vi "Get Specified FP Objects.vi"(8 "error in":errorcluster, 9 "Secondary Data":variant, 10 "Object Type":T1(ring)=enum."Generic", 11 "Diagram In":refnum<vi>) -> (0 "error out":errorcluster, 2 "All Objects":refnum<vi>[](array[refnum]), 3 "Diagram Out":refnum<vi>)   [LabVIEW 2012, in "Scripting Tools.lvlib"]
doc: "Returns all GObjects from the block diagram referenced by <B>Diagram In</B>, including all those in sub-diagrams (loops and sequence structures etc)."
uses:
  Scripting Tools.lvlib
  <vilib>/Utility/traverseref.llb/TRef TravTarget.ctl
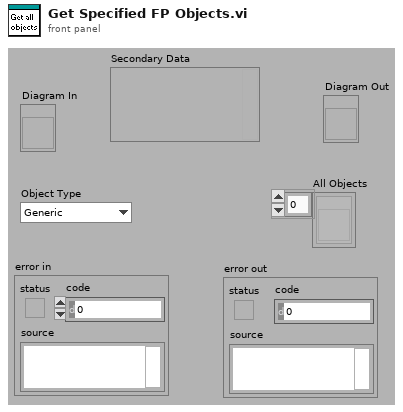
[diagram p1: front panel]
types:
  T1 = enum16{"Application", "VI", "PolymorphicVI", "MethodVI", "FacadeVI", "Generic", "FlatSequenceFrame", "TimeSequenceFrame", "SubWizard", "CodeWizard", "StateDiagramWizard", "MasterWizard", "Probe", "ConnectorPane", "Page", "Cursor", "Plot", "GObject", "TimedStructDCO", "SynchronousDataFlowDCO", "PolymorphicVISelector", "FlatSequenceOuterTunnel", "FlatSequenceInnerTunnel", "SimulationDCO", "FlatSequence", "TimeFlatSequence", "PropertyItem", "Wire", "SequenceLocal", "Tunnel", "SelectorTunnel", "LeftShiftRegister", "LoopTunnel", "RightShiftRegister", "Node", "TimedSequence", "XNode", "XDataNode", "StaticVIReference", "ControlReferenceConstant", "GrowableFunction", "Unbundler", "NamedUnbundler", "FormatScanString", "ObjectFunction", "Constructor", "Invoke", "Property", "CallLibrary", "CIN", "Bundler", "NamedBundler", "BuildArray", "IndexArray", "CompoundArithmetic", "BuildClusterArray", "Formula", "MathScriptNode", "ScriptNode", "Structure", "SynchronousDataFlowNode", "SimulationNode", "MultiFrameStructure", "DisableStructure", "EventStructure", "CaseStructure", "Sequence", "ExternalNode", "Loop", "WhileLoop", "TimedLoop", "ForLoop", "UnitCast", "CallByRef", "SubVI", "ConfNode", "PolymorphicSubVI", "Function", "FileDialog", "ArrayToCluster", "GPIBReadWrite", "FlattenUnflattenString", "FlattenString", "TypeCast", "ReadWriteFile", "Comparison", "Local", "Global", "FormulaParameter", "MathScriptNodeParameter", "ScriptNodeParameter", "Constant", "LabVIEWClassConstant", "AbsTimeConstant", "RefNumConstant", "ClassSpecifierConstant", "ColorBoxConstant", "IONameConstant", "GenClassTagFlatRefConstant", "GenClassTagRefConstant", "DAQmxNameConstant", "IVILogicalNameConstant", "VISAResourceNameConstant", "DAQChannelNameConstant", "DSCTagConstant", "BooleanConstant", "FixedConstant", "ClusterConstant", "StringConstant", "ComboBoxConstant", "NumericConstant", "NamedNumericConstant", "EnumConstant", "RingConstant", "DigitalNumericConstant", "ArrayConstant", "PathConstant", "Terminal", "OuterTerminal", "InnerTerminal", "ControlTerminal", "AbstractDiagram", "MathDiagram", "Diagram", "SDFCompanionDiagram", "SdfDiagram", "CompanionDiagram", "SimDiagram", "TopLevelDiagram", "Splitter", "Pane", "Scale", "SlideScale", "ColorGraphScale", "GraphScale", "ColorScale", "RotaryColorScale", "Panel", "Control", "LabVIEWClassControl", "SceneGraphDisplay", "Scrollbar", "Pixmap", "PlugInDDODummyContainer", "PlugInControl", "TreeControl", "SubPanel", "DigitalTable", "AbsTime", "PageSelector", "TabControl", "WaveformData", "MulticolumnListbox", "Cluster", "RadioButtonsControl", "IOName", "GenClassTagFlatRef", "GenClassTagRef", "DAQmxName", "IVILogicalName", "VISAResourceName", "DAQChannelName", "DSCTag", "String", "ComboBox", "GraphChart", "MixedSignalGraph", "IntensityGraph", "IntensityChart", "WaveformGraph", "DigitalGraph", "XYGraph", "WaveformChart", "Numeric", "NumericWithScale", "Knob", "Slide", "ColorRamp", "NamedNumeric", "Enum", "Ring", "Digital", "ActiveXContainer", "Picture", "Array", "Table", "ListBox", "Path", "LVVariant", "RefNum", "GenClassRef", "LVObjectRefNum", "VIRefNum", "TypedRefNum", "Boolean", "ColorBox", "Decoration", "Text", "NumericText", "Project", "ProjectItem", "PropertyFolder", "XPropertyFolder", "TargetItem", "Library", "XInterfaceLibrary", "XNodeLibrary", "XControlLibrary", "LVClassLibrary", "BuildSpecification", "Variable", "TagSet", "SceneWindow", "LVTarget", "Provider", "CopyOperation", "ProjectItemType", "CopyItem", "CopyConflict", "CopyExpert", "SceneNode", "SceneClipPlane", "SceneLight", "SceneObject", "SceneTexture", "SceneGeometry", "SceneMesh", "SceneSphere", "SceneHeightField", "SceneCylinder", "SceneCone", "SceneBox"}
  T2 = typedef "TRef TravTarget.ctl" = enum16{"FP", "BD", "Other"}
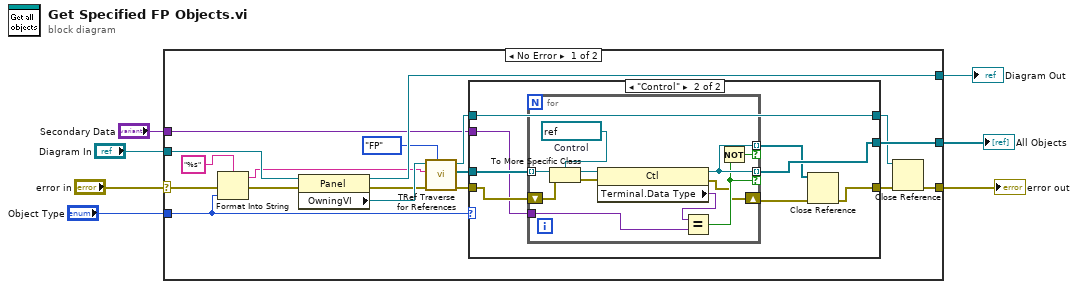
[diagram p0: block diagram]
diagram:
  n1 = case shown="No Error" "error in" {
    selector: "error in" -> [w9 w49]
    tunnel: [w22 w49] -> w7
    tunnel: "Diagram In" -> [w25 w48]
    tunnel: [w21 w48] -> w5
    tunnel: [w18 _] -> w3
    tunnel: "Secondary Data" -> [w13 _]
    tunnel: "Object Type" -> [w12 _]
    frame No Error {
      n2 = Format Into String(format string="%s", error in=w9, w12) -> (resulting string=w10:string, error out=w8:errorcluster)  [unwired: 1 in]
      n3 = property on="Property Node" class="Panel"(reference=w25, error in=w8) -> (reference out=w21:refnum<vi>, error out=w23:errorcluster, "OwningVI"=w24:refnum<vi>)
      n4 = call <vilib>:"TRef Traverse for References.vi"("Traverse Target"=TRef_TravTarget."FP", "error in (no error)"=w23, "Class Name"=w10, "VI Refnum"=w24) -> ("error out"=w14:errorcluster, "References"=w19:refnum<vi>[], "dup VI Refnum"=w16:refnum<vi>)  [unwired: 1 in, 4 out]
      n5 = case shown="\"Control\"" w12 {
        tunnel: w19 -> [w28 w35]
        tunnel: [w28 w32] -> w18
        tunnel: [w27 w36] -> w17
        tunnel: w16 -> [w27 w36]
        tunnel: [w26 w29] -> w15
        tunnel: w14 -> [w26 w34]
        tunnel: w13 -> [_ w33]
        frame "Generic", Default {
        }
        frame "Control" {
          n6 = for {
            tunnel: w35 -> [w47] mode=indexing
            shift-right: [w37] -> w31
            shift-left: w34 -> [w44]
            tunnel: w33 -> [w41]
            tunnel: [w40] -> w32 mode=indexing if=w39
            tunnel: [w40] -> w30 mode=indexing if=w38
            w46 = refnum<vi> refnum  # Control
            n7 = To More Specific Class(target class=w46, reference=w47, error in=w44) -> (specific class reference=w45:refnum<vi>, error out=w43:errorcluster)
            n8 = property class="Ctl"(reference=w45, error in=w43) -> (reference out=w40:refnum<vi>, error out=w37:errorcluster, "Terminal.Data Type"=w42:variant)
            n9 = Equal?(x=w42, y=w41) -> (x = y?=w39:bool)
            n10 = Not(x=w39) -> (.not. x?=w38:bool)
          }
          n11 = Close Reference(reference=w30, error in (no error)=w31) -> (error out=w29:errorcluster)
        }
      }
      n12 = Close Reference(reference=w17, error in (no error)=w15) -> (error out=w22:errorcluster)
    }
    frame Error {
    }
  }
  "error out" <- w7
  "All Objects" <- w3
  "Diagram Out" <- w5
